vi "Configure Jog.vi"(0 "VISA Resource Name":refnum<visa-resource-name>, 5 "Device Number (1)":i32=1, 7 "Enabled (False)":bool, 9 "Sensitivity (10)":i32=10, 11 "error in (no error)":errorcluster {"code" format="%.0x"}) -> (4 "VISA Resource Name Out":refnum<visa-resource-name>, 15 "error out":errorcluster {"code" format="%.0x"})   [LabVIEW 2018, in "Olympus IX BX Series.lvlib"]
doc: "Configures the jog operation."
uses:
  Olympus IX BX Series.lvlib
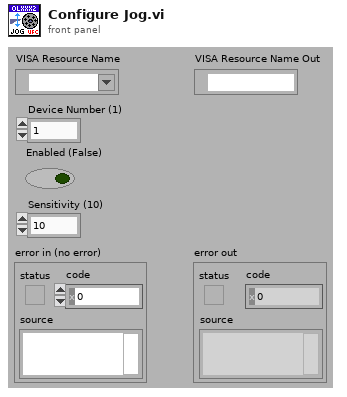
[diagram p1: front panel]
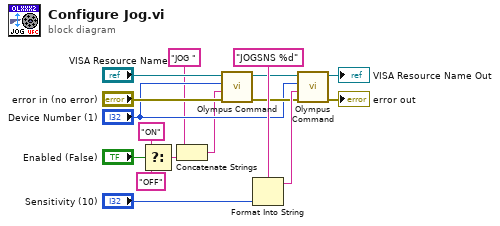
[diagram p0: block diagram]
diagram:
  n1 = Select(t="ON", s="Enabled (False)", f="OFF") -> (s? t:f=w4:string)
  n2 = Concatenate Strings("JOG " ("format string"), w4) -> (w2:string)
  n3 = call "Olympus Command.vi"("error in (no error)"="error in (no error)", "Command string"=w2, "Device Number (1)"="Device Number (1)", "VISA Resource Name"="VISA Resource Name") -> ("error out"=w10:errorcluster, "VISA Resource Name Out"=w9:refnum<visa-resource-name>)  [unwired: 5 in, 1 out]
  n4 = Format Into String(format string="JOGSNS %d", "Sensitivity (10)") -> (resulting string=w14:string)  [unwired: 2 in, 1 out]
  n5 = call "Olympus Command.vi"("error in (no error)"=w10, "Command string"=w14, "Device Number (1)"="Device Number (1)", "VISA Resource Name"=w9) -> ("error out"=→"error out":errorcluster, "VISA Resource Name Out"=→"VISA Resource Name Out":refnum<visa-resource-name>)  [unwired: 5 in, 1 out]
